vi "Control Bundle FPGA VI.vi"() -> ()   [LabVIEW 2011]
uses:
  <vilib>/Platform/TimedLoop/XDataNode/timing_clust.ctl
  <vilib>/Platform/TimedLoop/XDataNode/nitl_modes.ctl
  <vilib>/Platform/TimedLoop/XDataNode/wakeup.ctl
  <vilib>/rvi/eio/common/nirviEmuTemplateMethod_errors.vi
  <vilib>/Platform/TimedLoop/XDataNode/XDataNode.xnode
  <vilib>/eio/EIOMethodNode/EIOMethodNode.xnode
  <vilib>/eio/EIONode/EIONode.xnode
  <vilib>/Platform/TimedLoop/XDataNode/XDNodeRunTimeDep.lvlib
panel:
  in  "Mod3/DIO7":bool
  in  "Mod3/DIO6":bool
  in  "Mod3/DIO5":bool
  in  "Mod3/DIO4":bool
  out "Mod3/DIO3":bool
  out "Mod3/DIO2":bool
  out "Mod3/DIO1":bool
  out "Mod3/DIO0":bool
  in  "frequency (periods/tick) 3":fxp<+,32,0>
  in  "phase offset (periods) 3":fxp<+,32,0>
  in  "duty cycle (periods) 3":fxp<+,32,0>
  in  "frequency (periods/tick) 2":fxp<+,32,0>
  in  "phase offset (periods) 2":fxp<+,32,0>
  in  "duty cycle (periods) 2":fxp<+,32,0>
  in  "frequency (periods/tick) 1":fxp<+,32,0>
  in  "phase offset (periods) 1":fxp<+,32,0>
  in  "duty cycle (periods) 1":fxp<+,32,0>
  in  "duty cycle (periods) 0":fxp<+,32,0>
  in  "phase offset (periods) 0":fxp<+,32,0>
  in  "frequency (periods/tick) 0":fxp<+,32,0>
  in  "Reset Quad 0":bool
  in  "Reset Quad 1":bool
  out "Enc0 Pos (counts)":i32
  out "Enc1 Pos (counts)":i32
  in  "Mod2/AO3":fxp<+/-,20,5>
  in  "Mod2/AO2":fxp<+/-,20,5>
  in  "Mod2/AO1":fxp<+/-,20,5>
  in  "Mod2/AO0":fxp<+/-,20,5>
  out "Mod1/AI7":fxp<+/-,16,5>
  out "Mod1/AI6":fxp<+/-,16,5>
  out "Mod1/AI5":fxp<+/-,16,5>
  out "Mod1/AI4":fxp<+/-,16,5>
  out "Mod1/AI3":fxp<+/-,16,5>
  out "Mod1/AI2":fxp<+/-,16,5>
  out "Mod1/AI1":fxp<+/-,16,5>
  out "Mod1/AI0":fxp<+/-,16,5>
  # "Quadrature Encoder Input"
  # "PWM Generation"
  # "Digital  Output - Optional if PWM \nGeneration is disabled"
  # "Digital Input - Optional if Encoder \nInput is Disabled"
  # "Analog Out"
  # "Analog Input"
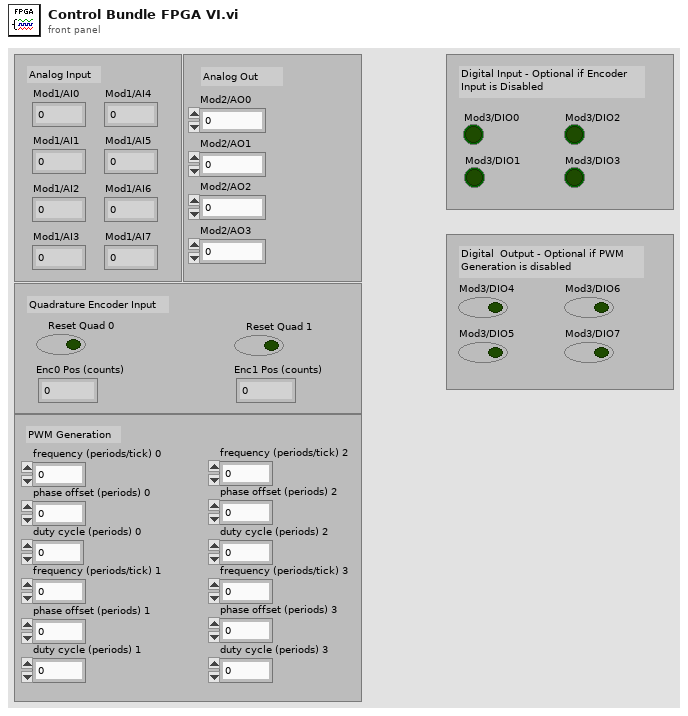
[diagram p1: front panel]
types:
  T1 = typedef "XDNodeRunTimeDep.lvlib/timing_clust.ctl" = cluster{"Expected End [f-1]":u64, "Actual End [f-1]":u64, "Finished Late? [f-1]":bool, "Expected End [i-1]":u64, "Actual End [i-1]":u64, "Finished Late? [i-1]":bool, "Expected Start [i]":u64, "Actual Start [i]":u64, "Expected Start [f]":u64, "Actual Start [f]":u64, "Source Name":string, "Structure Name":string, "Period":i64, "Deadline":i64, "Offset":i64, "Start":i64, "Priority":i32, "Timeout":i32, "Mode":T2, "Wakeup Reason":T3, "Error":errorcluster, "Source Type":string, "Secondary Source Type":string, "Global End Time":u64, "Global Start Time":u64, "Frame Duration":u64, "Iteration Duration":u64, "Assigned CPU":i32, "I/O Scan Engine Mode":u32}
  T2 = typedef "XDNodeRunTimeDep.lvlib/nitl_modes.ctl" = enum32{"No Change", "Process missed periods, maintain original phase", "Discard missed periods, maintain original phase", "Process missed periods, ignore original phase", "Discard missed periods, ignore original phase"}
  T3 = typedef "XDNodeRunTimeDep.lvlib/wakeup.ctl" = enum32{"Normal", "Aborted", "Asynchronous wakeup", "Timing source error", "Timed loop error", "Timeout"}
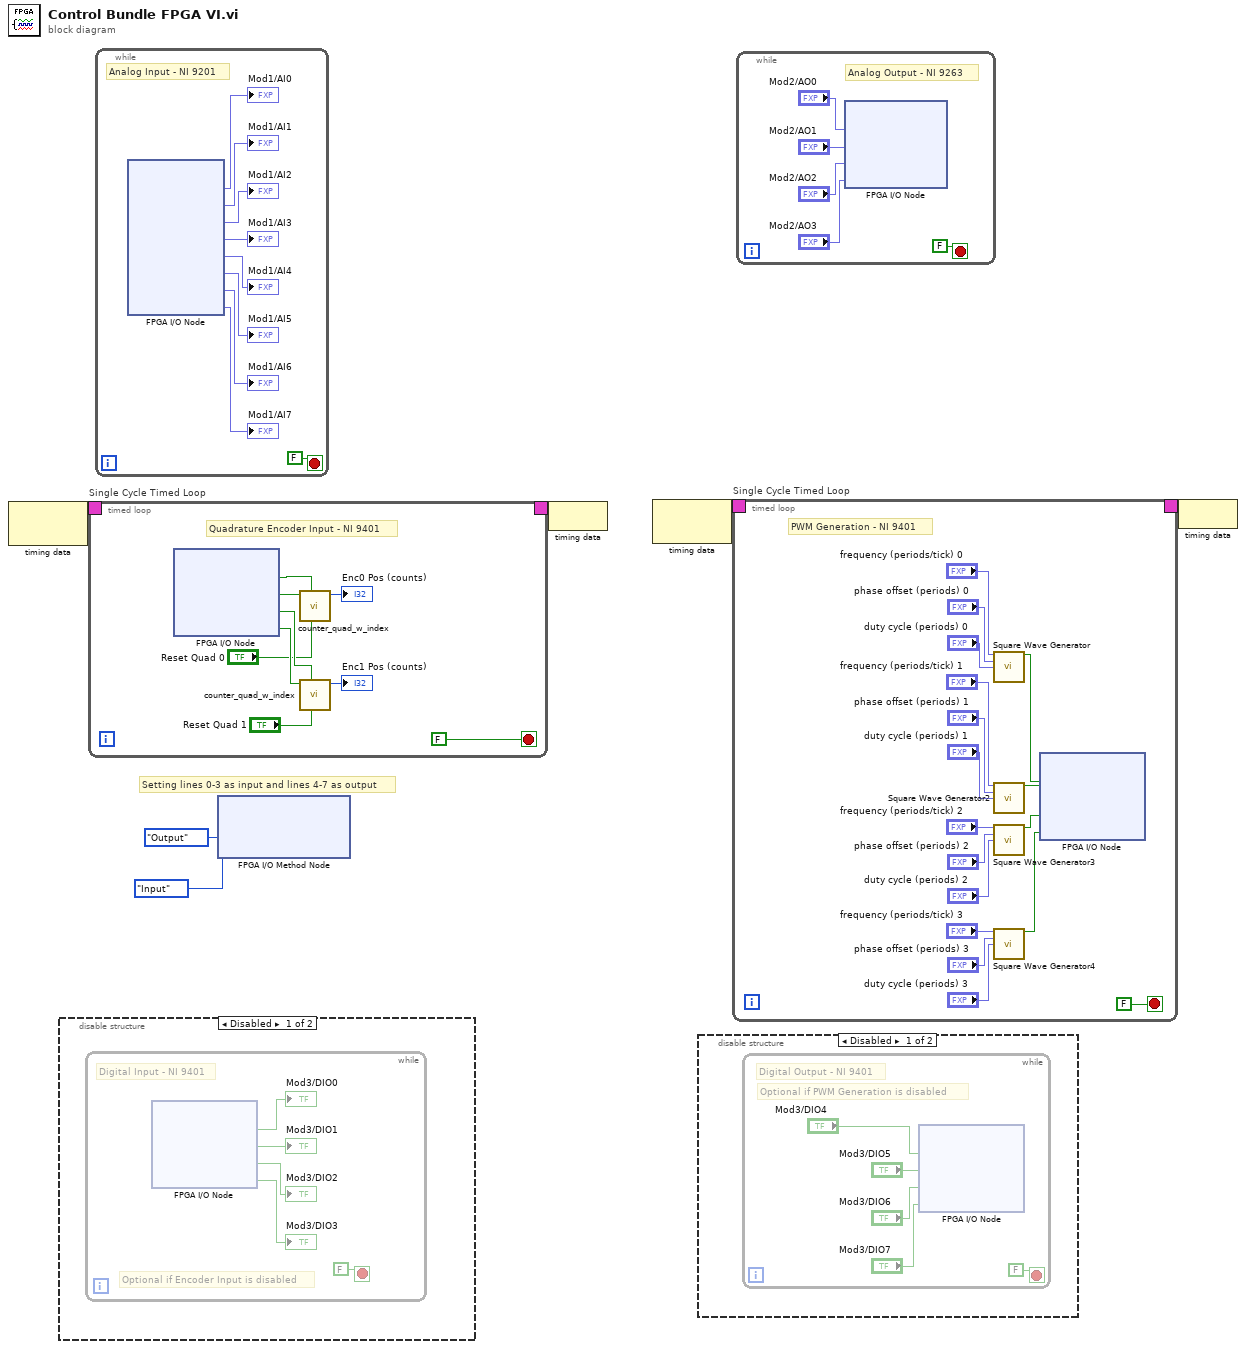
[diagram p0: block diagram]
diagram:
  # "Setting lines 0-3 as input and lines 4-7 as output"
  n1 = node-c288() -> (w4:T1)  [unwired: 1 in]
  n2 = disable-structure shown="Disabled" {
    frame Disabled {
      n3 = while {
        stop <- FALSE stop-if-true
        # "Optional if Encoder Input is disabled"
        # "Digital Input - NI 9401"
        n4 = xnode "FPGA I/O Node"() -> ("Mod3/DIO0"=→"Mod3/DIO0":bool, "Mod3/DIO1"=→"Mod3/DIO1":bool, "Mod3/DIO2"=→"Mod3/DIO2":bool, "Mod3/DIO3"=→"Mod3/DIO3":bool)  [unwired: 4 in, 4 out]
      }
    }
    frame Enabled {
    }
  }
  n5 = timed-loop "Single Cycle Timed Loop" {
    timing: w4 -> [_]
    timing-out: [_] -> w3
    stop <- FALSE stop-if-true
    # "Quadrature Encoder Input - NI 9401"
    n6 = xnode "FPGA I/O Node"() -> ("Mod3/DIO0"=w16:bool, "Mod3/DIO1"=w15:bool, "Mod3/DIO2"=w14:bool, "Mod3/DIO3"=w13:bool)  [unwired: 4 in, 4 out]
    n7 = call "counter_quad_w_index.vi"("Reset"="Reset Quad 0", "A"=w16, "B"=w15) -> ("Position (counts)"=→"Enc0 Pos (counts)":i32)  [unwired: 8 in]
    n8 = call "counter_quad_w_index.vi"("Reset"="Reset Quad 1", "A"=w14, "B"=w13) -> ("Position (counts)"=→"Enc1 Pos (counts)":i32)  [unwired: 8 in]
  }
  n9 = while {
    stop <- FALSE stop-if-true
    # "Analog Input - NI 9201"
    n10 = xnode "FPGA I/O Node"() -> ("Mod1/AI0"=→"Mod1/AI0":fxp<+/-,16,5>, "Mod1/AI1"=→"Mod1/AI1":fxp<+/-,16,5>, "Mod1/AI2"=→"Mod1/AI2":fxp<+/-,16,5>, "Mod1/AI3"=→"Mod1/AI3":fxp<+/-,16,5>, "Mod1/AI4"=→"Mod1/AI4":fxp<+/-,16,5>, "Mod1/AI5"=→"Mod1/AI5":fxp<+/-,16,5>, "Mod1/AI6"=→"Mod1/AI6":fxp<+/-,16,5>, "Mod1/AI7"=→"Mod1/AI7":fxp<+/-,16,5>)  [unwired: 8 in, 8 out]
  }
  n11 = xnode "FPGA I/O Method Node"("DIO 7:4"=enum8{"No Change", "Input", "Output"}."Output", "DIO 3:0"=enum8{"No Change", "Input", "Output"}."Input") -> ()  [unwired: 1 in, 1 out]
  n12 = node-c288(w3) -> ()
  n13 = node-c288() -> (w6:T1)  [unwired: 1 in]
  n14 = disable-structure shown="Disabled" {
    frame Disabled {
      n15 = while {
        stop <- FALSE stop-if-true
        # "Optional if PWM Generation is disabled"
        # "Digital Output - NI 9401"
        n16 = xnode "FPGA I/O Node"("Mod3/DIO4"="Mod3/DIO4", "Mod3/DIO5"="Mod3/DIO5", "Mod3/DIO6"="Mod3/DIO6", "Mod3/DIO7"="Mod3/DIO7") -> ()  [unwired: 4 in, 4 out]
      }
    }
    frame Enabled {
    }
  }
  n17 = timed-loop "Single Cycle Timed Loop" {
    timing: w6 -> [_]
    timing-out: [_] -> w5
    stop <- FALSE stop-if-true
    # "PWM Generation - NI 9401"
    n18 = call "Square Wave Generator"("frequency (periods/tick)"="frequency (periods/tick) 0", "phase offset (periods)"="phase offset (periods) 0", "duty cycle (periods)"="duty cycle (periods) 0") -> ("square wave out"=w50:bool)  [unwired: 12 in]
    n19 = call "Square Wave Generator2"("frequency (periods/tick)"="frequency (periods/tick) 1", "phase offset (periods)"="phase offset (periods) 1", "duty cycle (periods)"="duty cycle (periods) 1") -> ("square wave out"=w40:bool)  [unwired: 12 in]
    n20 = call "Square Wave Generator3"("frequency (periods/tick)"="frequency (periods/tick) 2", "phase offset (periods)"="phase offset (periods) 2", "duty cycle (periods)"="duty cycle (periods) 2") -> ("square wave out"=w39:bool)  [unwired: 12 in]
    n21 = call "Square Wave Generator4"("frequency (periods/tick)"="frequency (periods/tick) 3", "phase offset (periods)"="phase offset (periods) 3", "duty cycle (periods)"="duty cycle (periods) 3") -> ("square wave out"=w38:bool)  [unwired: 12 in]
    n22 = xnode "FPGA I/O Node"("Mod3/DIO4"=w50, "Mod3/DIO5"=w40, "Mod3/DIO6"=w39, "Mod3/DIO7"=w38) -> ()  [unwired: 4 in, 4 out]
  }
  n23 = while {
    stop <- FALSE stop-if-true
    # "Analog Output - NI 9263"
    n24 = xnode "FPGA I/O Node"("Mod2/AO0"="Mod2/AO0", "Mod2/AO1"="Mod2/AO1", "Mod2/AO2"="Mod2/AO2", "Mod2/AO3"="Mod2/AO3") -> ()  [unwired: 4 in, 4 out]
  }
  n25 = node-c288(w5) -> ()
